vi "Arcade Drive.vi"(2 "Throttle":dbl, 3 "Turn":dbl) -> (0 "Right Motors":dbl, 1 "Left Motors":dbl)   [LabVIEW 2015]
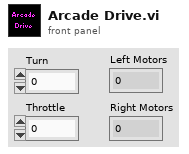
[diagram p1: front panel]
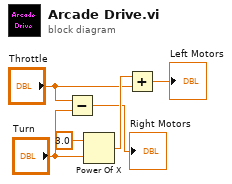
[diagram p0: block diagram]
diagram:
  n1 = Subtract(x="Throttle", y="Turn") -> (x-y=→"Right Motors":dbl)
  n2 = Power Of X(1:"Turn", 2:3.0 ("y")) -> (0:w5:dbl)
  n3 = Add(x=w5, y="Throttle") -> (x+y=→"Left Motors":dbl)
